vi "子界面-查看某框-只读穿透图模式.vi"(0 "框号":dbl format="%#_13g", 1 "框组":T3(array[cluster]), 2 "临界Z值":i32, 4 "临界面积百分比值":dbl, 5 "预先配置的灰度阈值":dbl, 6 "穿透图原始路径":path, 7 "部位信息":string[](array[string])=["", "34.500000", "32.500000", "1121", "34", "54.955926", "分层类", "不合格", ""], 12 "产品规格":cluster{"产品长度（周长）（mm）":dbl, "产品宽度（母线长）（mm）":dbl}) -> (14 "弥散类检测结果":string[][](table), 19 "分层类检测结果":string[][](table))   [LabVIEW 2018]
uses:
  <vilib>/vision/NI_Vision_Development_Module.lvlib
panel:
  in  "Tab Control":T1
  out "?":T2(plugin-control)
  out "Threshold Image":T2(plugin-control)
  out "Threshold Image":T2(plugin-control)
  in  "格式字符串 3":string="%f"
  in  "分隔符（'\\'代码显示） 2":string="\t"
  out "弥散和分层临界灰度值":i64
  out "弥散缺陷个数":i32
  out "分层缺陷个数":i32
  out "合格？ 弥散类":string="fencengThreshold"
  out "合格？分层类":string="fencengThreshold"
  in  "stop":bool caption="停止"
  out "弥散测量结果":dbl[][](array[numeric]) format="%.2f"
  out "?":string
  out "面积 (pixels)":i32
  in  "格式字符串 2":string="%f"
  in  "分隔符（'\\'代码显示）":string="\t"
  out "分层测量结果":dbl[][](array[numeric]) format="%.2f"
  out "缺陷初步分类的临界值":sgl format="%#.3f"
  # "所选区域信息"
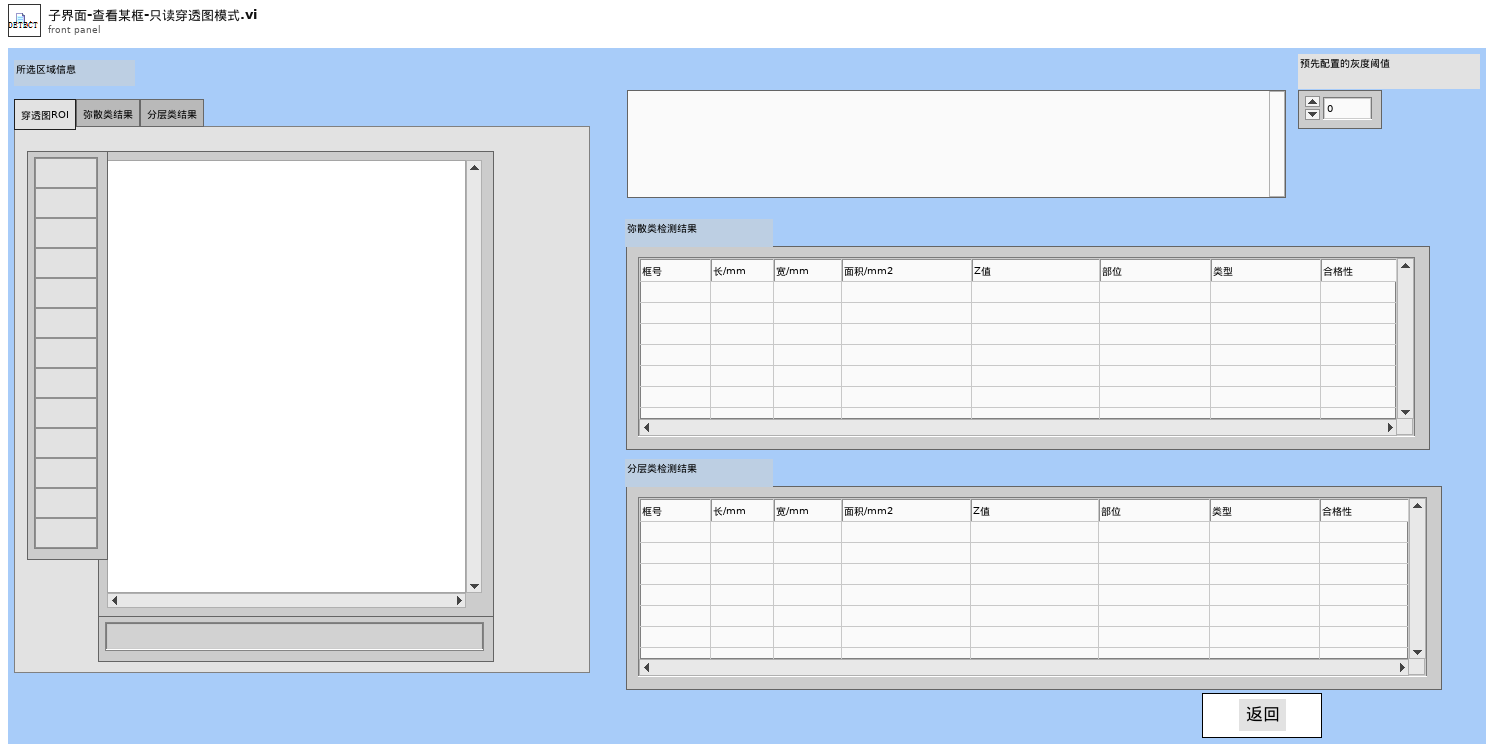
[diagram p1: front panel]
types:
  T1 = typedef "控件2.ctl" = enum32{"穿透图ROI", "弥散类结果", "分层类结果"}
  T2 = typedef "IMAQ Image.ctl" = refnum<image>
  T3 = cluster{"Global Rectangle":i32[], "Contours":cluster{"Contour Type":u32, "ROI Type":u32, "Points":i32[]}[]}[]
  T4 = typedef "Image Type" = u32
  T5 = typedef "Particle Parameters" = i32
  T6 = cluster{"Measurement Parameter":T5, "Range Lower Value":dbl, "Range Upper Value":dbl, "Range":bool, "Measurement Type":bool}[]
  T7 = cluster{"Global Rectangle":i32[], "Contours":cluster{"Contour Type":u32, "ROI Type":u32, "Points":i32[]}[]}
  T8 = cluster{"histogram":u32[], "Minimal Value":sgl, "Maximal Value":sgl, "Starting Value":sgl, "Interval Width":sgl, "Mean Value":sgl, "Standard  Variation":sgl, "Area (pixels)":i32}
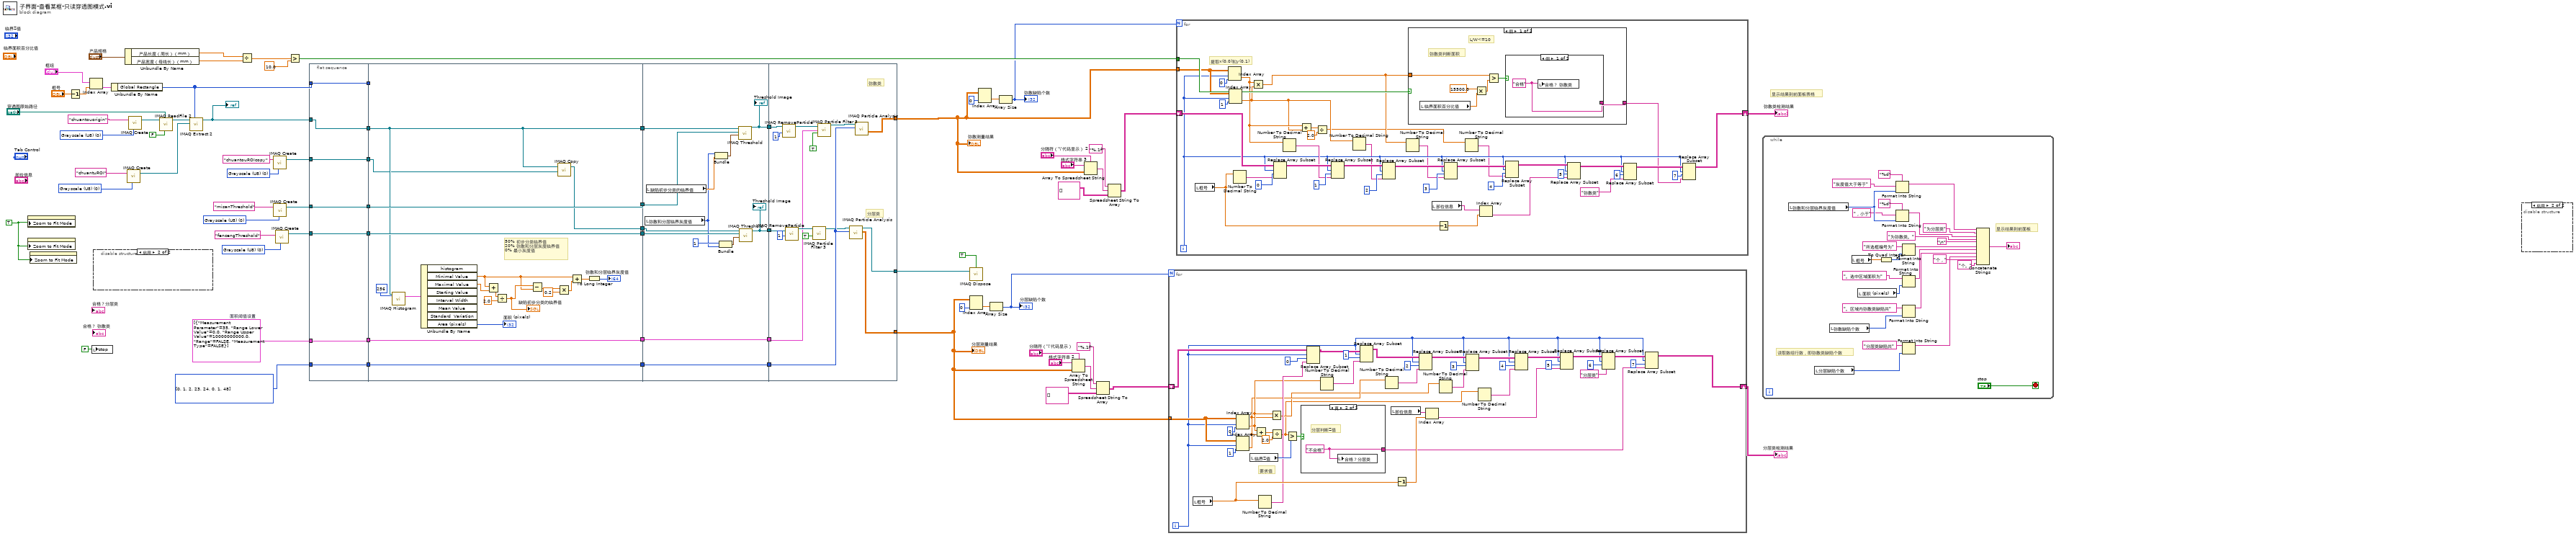
[diagram p0: block diagram]
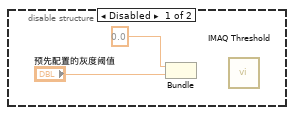
[diagram p2: hidden frame]
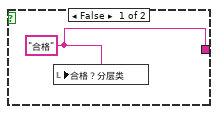
[diagram p3: hidden frame]
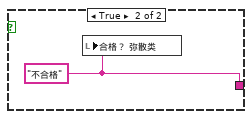
[diagram p4: hidden frame]
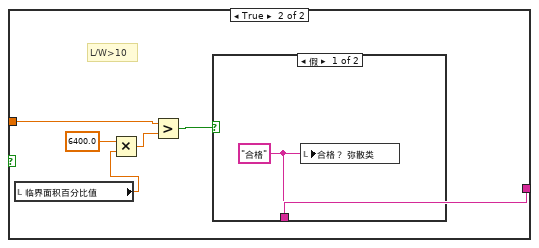
[diagram p5: hidden frame]
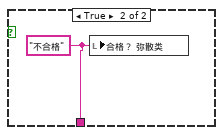
[diagram p6: hidden frame]
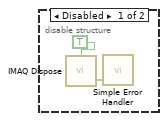
[diagram p7: hidden frame]
diagram:
  w1 = T4 0 items=["Grayscale (U8)", "Grayscale (I16)", "Grayscale (SGL)", "Complex (CSG)", "RGB (U32)", "HSL (U32)", "RGB (U64)", "Grayscale (U16)"] ("Image Type")
  w6 = TRUE ("Zoom to Fit Mode")
  w51 = T4 0 items=["Grayscale (U8)", "Grayscale (I16)", "Grayscale (SGL)", "Complex (CSG)", "RGB (U32)", "HSL (U32)", "RGB (U64)", "Grayscale (U16)"] ("Image Type")
  w52 = T4 0 items=["Grayscale (U8)", "Grayscale (I16)", "Grayscale (SGL)", "Complex (CSG)", "RGB (U32)", "HSL (U32)", "RGB (U64)", "Grayscale (U16)"] ("Image Type")
  w55 = T4 0 items=["Grayscale (U8)", "Grayscale (I16)", "Grayscale (SGL)", "Complex (CSG)", "RGB (U32)", "HSL (U32)", "RGB (U64)", "Grayscale (U16)"] ("Image Type")
  w29 = i32[] [0, 1, 2, 23, 24, 0, 1, 48] items=["Bounding Rect Width", "Bounding Rect Height", "Area"] ("Pixel Measurements")
  w33 = T6 [{"Measurement Parameter"=35, "Range Lower Value"=0.0, "Range Upper Value"=10000000000.0, "Range"=FALSE, "Measurement Type"=FALSE}]  # 面积阈值设置
  w70 = T4 0 items=["Grayscale (U8)", "Grayscale (I16)", "Grayscale (SGL)", "Complex (CSG)", "RGB (U32)", "HSL (U32)", "RGB (U64)", "Grayscale (U16)"] ("Image Type")
  # "显示结果到前面板表格"
  n1 = property class="ImageControl"("Zoom to Fit Mode"=w6) -> ()  [unwired: 2 in, 2 out]
  n2 = property class="ImageControl"("Zoom to Fit Mode"=w6) -> ()  [unwired: 2 in, 2 out]
  n3 = property class="ImageControl"("Zoom to Fit Mode"=w6) -> ()  [unwired: 2 in, 2 out]
  n4 = Decrement(x="框号") -> (x-1=w72:dbl)
  n5 = Index Array(array="框组", index=w72) -> (element=w73:T7)
  n6 = local write "stop"(FALSE ("stop")) -> ()
  n7 = disable-structure shown="启用" {
    frame Disabled {
      n8 = Bundle(0.0, "预先配置的灰度阈值"="预先配置的灰度阈值") -> ()  [unwired: 1 in, 1 out]
      n9 = call "IMAQ Threshold"() -> ()  [unwired: 6 in, 6 out]
    }
    frame Enabled {
    }
  }
  n10 = Unbundle By Name(w73) -> ("Global Rectangle"=w45:i32[])
  n11 = Unbundle By Name("产品规格") -> ("产品长度（周长）（mm）"=w63:dbl, "产品宽度（母线长）（mm）"=w62:dbl)
  n12 = call "IMAQ Create"("Image Name"="chuantuROI", "Image Type"=w55) -> ("New Image"=w54:T2)  [unwired: 3 in, 1 out]
  n13 = call "IMAQ Create"("Image Name"="chuantouorigin", "Image Type"=w70) -> ("New Image"=w57:T2)  [unwired: 3 in, 1 out]
  n14 = call "IMAQ ReadFile 2"("Use File Path Image Type"=FALSE, "File Path"="穿透图原始路径", "Image"=w57) -> ("Image Out"=w58:T2)  [unwired: 4 in, 4 out]
  n15 = call "IMAQ Extract 2"("Optional Rectangle"=w45, "Image Dst"=w54, "Image Src"=w58) -> ("Image Dst Out"=w9:T2)  [unwired: 7 in, 1 out]
  "?" <- w9
  n16 = Divide(x=w63, y=w62) -> (x/y=w66:dbl)
  n17 = call "IMAQ Create"("Image Name"="chuantouROIcopy", "Image Type"=w1) -> ("New Image"=w4:T2)  [unwired: 3 in, 1 out]
  n18 = call "IMAQ Create"("Image Name"="misanThreshold", "Image Type"=w51) -> ("New Image"=w41:T2)  [unwired: 3 in, 1 out]
  n19 = call "IMAQ Create"("Image Name"="fencengThreshold", "Image Type"=w52) -> ("New Image"=w39:T2)  [unwired: 3 in, 1 out]
  n20 = Greater?(x=w66, y=10.0) -> (0:w61:bool)
  n21 = flat-sequence {
    tunnel: w45 -> [w84]
    tunnel: w9 -> [w79]
    tunnel: [w84] -> w44
    tunnel: w41 -> [w83]
    tunnel: [w83] -> w42
    tunnel: [w82] -> w40
    tunnel: w39 -> [w82]
    tunnel: [w81] -> w34
    tunnel: w33 -> [w81]
    tunnel: [w80] -> w30
    tunnel: w29 -> [w80]
    tunnel: [w79] -> w7
    tunnel: w4 -> [w78]
    tunnel: [w78] -> w3
    tunnel: [w104] -> w43
    tunnel: [w103] -> w38
    tunnel: [w98] -> w32
    tunnel: [w97] -> w28
    tunnel: w30 -> [w97]
    tunnel: w34 -> [w98]
    tunnel: w40 -> [w103]
    tunnel: w42 -> [w104]
    tunnel: w44 -> [_]
    tunnel: [w87] -> w8
    tunnel: w7 -> [w87]
    tunnel: [w86] -> w5
    tunnel: w3 -> [w85]
    tunnel: w43 -> [w117]
    tunnel: w38 -> [w116]
    tunnel: [w106] -> w36
    tunnel: [w107] -> w35
    tunnel: w32 -> [w115]
    tunnel: [w115] -> w31
    tunnel: w28 -> [w114]
    tunnel: [w114] -> w27
    tunnel: w8 -> [w108]
    tunnel: w5 -> [w105]
    tunnel: [w129] -> w12
    tunnel: [w125] -> w20
    tunnel: [w124] -> w37
    tunnel: w36 -> [w123]
    tunnel: w35 -> [w122]
    tunnel: w31 -> [w121]
    tunnel: w27 -> [w120]
    frame #0 {
    }
    frame #1 {
      # "50% 初步分类临界值\n20% 弥散和分层灰度临界值\n0% 最小灰度值"
      n22 = call "IMAQ Histogram"("Number of Classes"=256, "Image"=w87) -> ("Histogram Report"=w101:T8)  [unwired: 8 in, 1 out]
      n23 = Unbundle By Name(w101) -> ("Minimal Value"=w89:sgl, "Maximal Value"=w95:sgl, "Area (pixels)"=→"面积 (pixels)":i32)  [unwired: 5 out]
      n24 = Add(x=w89, y=w95) -> (x+y=w94:sgl)
      n25 = Divide(x=w94, y=sgl 2.0) -> (x/y=w93:sgl)
      "缺陷初步分类的临界值" <- w93
      n26 = Subtract(x=w93, y=w89) -> (x-y=w91:sgl)
      n27 = Multiply(x=w91, y=0.2) -> (x*y=w90:dbl)
      n28 = call "IMAQ Copy"("Image Dst"=w85, "Image Src"=w87) -> ("Image Dst Out"=w86:T2)  [unwired: 4 in, 1 out]
      n29 = Add(x=w89, y=w90) -> (x+y=w88:dbl)
      n30 = To Long Integer(number=w88) -> (32bit integer=→"弥散和分层临界灰度值":i32)
    }
    frame #2 {
      n31 = local read "弥散和分层临界灰度值"() -> (w110:i64)
      n32 = local read "缺陷初步分类的临界值"() -> (w112:sgl)
      n33 = Bundle("弥散和分层临界灰度值"=w110, "缺陷初步分类的临界值"=w112) -> (w113:cluster{"弥散和分层临界灰度值":i64, "缺陷初步分类的临界值":sgl})  [unwired: 1 in]
      n34 = Bundle(1, "弥散和分层临界灰度值"=w110) -> (w109:cluster{i32, "弥散和分层临界灰度值":i64})  [unwired: 1 in]
      n35 = call "IMAQ Threshold"("Range"=w113, "Image Dst"=w117, "Image Src"=w108) -> ("Image Dst Out"=w107:T2)  [unwired: 3 in, 5 out]
      "Threshold Image" <- w107
      n36 = call "IMAQ Threshold"("Range"=w109, "Image Dst"=w116, "Image Src"=w105) -> ("Image Dst Out"=w106:T2)  [unwired: 3 in, 5 out]
      "Threshold Image" <- w106
    }
    frame #3 {
      # "分层类"
      # "弥散类"
      n37 = call "IMAQ RemoveParticle"("Number of Erosion"=1, "Image Src"=w122) -> ("Image Dst Out"=w132:T2)  [unwired: 8 in, 1 out]
      n38 = call "IMAQ RemoveParticle"("Number of Erosion"=1, "Image Src"=w123) -> ("Image Dst Out"=w128:T2)  [unwired: 8 in, 1 out]
      n39 = call "IMAQ Particle Filter 3"("Image Src"=w128, "Keep/Remove Particles (F)"=TRUE) -> ("Image Dst Out"=w118:T2)  [unwired: 11 in, 2 out]
      n40 = call "IMAQ Particle Filter 3"("Image Src"=w132, "Selection Values"=w121, "Keep/Remove Particles (F)"=TRUE) -> ("Image Dst Out"=w119:T2)  [unwired: 10 in, 2 out]
      n41 = call "IMAQ Particle Analysis"("Pixel Measurements"=w120, "Image"=w118) -> ("Particle Measurements (Pixels)"=w125:dbl[][], "Image Out (duplicate)"=w124:T2)  [unwired: 4 in, 4 out]
      n42 = call "IMAQ Particle Analysis"("Pixel Measurements"=w120, "Image"=w119) -> ("Particle Measurements (Real-World)"=w129:dbl[][])  [unwired: 4 in, 5 out]
    }
  }
  n43 = call "IMAQ Dispose"("All Images? (No)"=TRUE, "Image"=w37) -> ()  [unwired: 4 in, 1 out]
  n44 = Index Array(array=w20, index (col)=0 ("禁用的索引 (列)")) -> (element=w49:dbl[])  [unwired: 1 in]
  n45 = Index Array(array=w12, index (col)=0 ("禁用的索引 (列)")) -> (element=w47:dbl[])  [unwired: 1 in]
  n46 = Array Size(array=w49) -> (size(s)=w26:i32)
  "分层缺陷个数" <- w26
  n47 = Array Size(array=w47) -> (size(s)=w60:i32)
  "弥散缺陷个数" <- w60
  n48 = Array To Spreadsheet String(delimiter (Tab)="分隔符（'\\'代码显示）", array=w20, 3:"格式字符串 2") -> (spreadsheet string=w23:string)
  n49 = Array To Spreadsheet String(delimiter (Tab)="分隔符（'\\'代码显示） 2", array=w12, 3:"格式字符串 3") -> (spreadsheet string=w15:string)
  n50 = Spreadsheet String To Array(format string="%.1f", spreadsheet string=w23, array type (2D Dbl)=string[][] [] ("Array")) -> (array=w19:string[][])  [unwired: 1 in]
  n51 = Spreadsheet String To Array(format string="%.1f", spreadsheet string=w15, array type (2D Dbl)=string[][] [] ("Array")) -> (array=w11:string[][])  [unwired: 1 in]
  n52 = for {
    N: w26 -> [_]
    tunnel: w20 -> [w164]
    shift-right: [w142] -> w18
    shift-left: w19 -> [w153]
    i -> [w137]
    # "要求值"
    n53 = local read "框号"() -> (w162:dbl)
    n54 = Index Array(array=w164, index (row)=w137, index (col)=0 ("禁用的索引 (列)")) -> (element=w141:dbl)
    n55 = Index Array(array=w164, index (row)=w137, index (col)=1 ("禁用的索引 (列)")) -> (element=w140:dbl)
    n56 = local read "临界Z值"() -> (w170:i32)
    n57 = Add(x=w141, y=w140) -> (x+y=w171:dbl)
    n58 = Number To Decimal String(number=w162) -> (decimal integer string=w154:string)  [unwired: 1 in]
    n59 = Multiply(x=w141, y=w140) -> (x*y=w139:dbl)
    n60 = Divide(x=w171, y=2.0) -> (x/y=w136:dbl)
    n61 = Greater?(x=w136, y=w170) -> (0:w172:bool)
    n62 = case shown="真" w172 {
      tunnel: [w173 w174] -> w133
      frame False {
        w173 = "合格" ("合格？")
        n63 = local write "合格？分层类"(w173) -> ()
      }
      frame True {
        w174 = "不合格" ("合格？")
        # "分层判断Z值"
        n64 = local write "合格？分层类"(w174) -> ()
      }
    }
    n65 = Replace Array Subset(array=w153, new element=w154, index (row)=w137, index (col)=0 ("索引 (列)")) -> (w152:string[][])
    n66 = Number To Decimal String(number=w141) -> (decimal integer string=w151:string)  [unwired: 1 in]
    n67 = Replace Array Subset(array=w152, new element=w151, index (row)=w137, index (col)=1 ("索引 (列)")) -> (w149:string[][])
    n68 = Number To Decimal String(number=w140) -> (decimal integer string=w150:string)  [unwired: 1 in]
    n69 = local read "部位信息"() -> (w166:string[])
    n70 = Decrement(x=w162) -> (x-1=w165:dbl)
    n71 = Replace Array Subset(array=w149, new element=w150, index (row)=w137, index (col)=2 ("索引 (列)")) -> (w148:string[][])
    n72 = Index Array(array=w166, index=w165) -> (element=w135:string)
    n73 = Number To Decimal String(number=w139) -> (decimal integer string=w147:string)  [unwired: 1 in]
    n74 = Replace Array Subset(array=w148, new element=w147, index (row)=w137, index (col)=3 ("索引 (列)")) -> (w146:string[][])
    n75 = Number To Decimal String(number=w136) -> (decimal integer string=w138:string)  [unwired: 1 in]
    n76 = Replace Array Subset(array=w146, new element=w138, index (row)=w137, index (col)=4 ("索引 (列)")) -> (w145:string[][])
    n77 = Replace Array Subset(array=w145, new element=w135, index (row)=w137, index (col)=5 ("索引 (列)")) -> (w144:string[][])
    n78 = Replace Array Subset(array=w144, new element="分层类" ("新元素/子数组"), index (row)=w137, index (col)=6 ("索引 (列)")) -> (w143:string[][])
    n79 = Replace Array Subset(array=w143, new element=w133, index (row)=w137, index (col)=7 ("索引 (列)")) -> (w142:string[][])
  }
  "分层类检测结果" <- w18
  n80 = for {
    N: w60 -> [_]
    tunnel: w61 -> [w213]
    tunnel: w12 -> [w212]
    shift-right: [w192] -> w10
    shift-left: w11 -> [w200]
    i -> [w190]
    # "提取x(0,0)和y(0,1)"
    n81 = local read "框号"() -> (w178:dbl)
    n82 = Index Array(array=w212, index (row)=w190, index (col)=0 ("禁用的索引 (列)")) -> (element=w184:dbl)
    n83 = Index Array(array=w212, index (row)=w190, index (col)=1 ("禁用的索引 (列)")) -> (element=w183:dbl)
    n84 = Number To Decimal String(number=w178) -> (decimal integer string=w201:string)  [unwired: 1 in]
    n85 = Multiply(x=w184, y=w183) -> (x*y=w188:dbl)
    n86 = Replace Array Subset(array=w200, new element=w201, index (row)=w190, index (col)=0 ("索引 (列)")) -> (w199:string[][])
    n87 = Number To Decimal String(number=w184) -> (decimal integer string=w191:string)  [unwired: 1 in]
    n88 = Add(x=w184, y=w183) -> (x+y=w186:dbl)
    n89 = Divide(x=w186, y=2.0) -> (x/y=w182:dbl)
    n90 = Replace Array Subset(array=w199, new element=w191, index (row)=w190, index (col)=1 ("索引 (列)")) -> (w198:string[][])
    n91 = Number To Decimal String(number=w183) -> (decimal integer string=w189:string)  [unwired: 1 in]
    n92 = Replace Array Subset(array=w198, new element=w189, index (row)=w190, index (col)=2 ("索引 (列)")) -> (w197:string[][])
    n93 = Number To Decimal String(number=w188) -> (decimal integer string=w187:string)  [unwired: 1 in]
    n94 = case shown="假" w213 {
      tunnel: w188 -> [w219 w227]
      tunnel: [w217 w225] -> w175
      frame False {
        # "弥散类判断面积"
        # "L/W<=10"
        n95 = local read "临界面积百分比值"() -> (w215:dbl)
        n96 = Multiply(x=15500.0, y=w215) -> (x*y=w214:dbl)
        n97 = Greater?(x=w219, y=w214) -> (0:w218:bool)
        n98 = case shown="假" w218 {
          tunnel: [w220 w221] -> w217
          frame False {
            w220 = "合格" ("合格？")
            n99 = local write "合格？ 弥散类"(w220) -> ()
          }
          frame True {
            w221 = "不合格" ("合格？")
            n100 = local write "合格？ 弥散类"(w221) -> ()
          }
        }
      }
      frame True {
        # "L/W>10"
        n101 = local read "临界面积百分比值"() -> (w222:dbl)
        n102 = Multiply(x=6400.0, y=w222) -> (x*y=w224:dbl)
        n103 = Greater?(x=w227, y=w224) -> (0:w226:bool)
        n104 = case shown="假" w226 {
          tunnel: [w228 w229] -> w225
          frame False {
            w228 = "合格" ("合格？")
            n105 = local write "合格？ 弥散类"(w228) -> ()
          }
          frame True {
            w229 = "不合格" ("合格？")
            n106 = local write "合格？ 弥散类"(w229) -> ()
          }
        }
      }
    }
    n107 = local read "部位信息"() -> (w180:string[])
    n108 = Decrement(x=w178) -> (x-1=w179:dbl)
    n109 = Replace Array Subset(array=w197, new element=w187, index (row)=w190, index (col)=3 ("索引 (列)")) -> (w196:string[][])
    n110 = Number To Decimal String(number=w182) -> (decimal integer string=w181:string)  [unwired: 1 in]
    n111 = Index Array(array=w180, index=w179) -> (element=w177:string)
    n112 = Replace Array Subset(array=w196, new element=w181, index (row)=w190, index (col)=4 ("索引 (列)")) -> (w195:string[][])
    n113 = Replace Array Subset(array=w195, new element=w177, index (row)=w190, index (col)=5 ("索引 (列)")) -> (w194:string[][])
    n114 = Replace Array Subset(array=w194, new element="弥散类" ("新元素/子数组"), index (row)=w190, index (col)=6 ("索引 (列)")) -> (w193:string[][])
    n115 = Replace Array Subset(array=w193, new element=w175, index (row)=w190, index (col)=7 ("索引 (列)")) -> (w192:string[][])
  }
  "弥散类检测结果" <- w10
  n116 = while {
    stop <- "stop" stop-if-true
    # "显示结果到前面板"
    # "读取数组行数，即弥散类缺陷个数"
    n117 = local read "弥散和分层临界灰度值"() -> (w256:i64)
    n118 = local read "分层缺陷个数"() -> (w231:i32)
    n119 = local read "弥散缺陷个数"() -> (w230:i32)
    n120 = local read "框号"() -> (w247:dbl)
    n121 = local read "面积 (pixels)"() -> (w250:i32)
    n122 = To Quad Integer(1:w247) -> (0:w248:i64)
    n123 = Format Into String(format string="%d" ("格式字符串"), initial string="灰度值大于等于" ("初始字符串"), w256) -> (resulting string=w252:string)  [unwired: 1 in, 1 out]
    n124 = Format Into String(format string="%d" ("格式字符串"), initial string="，小于" ("初始字符串"), w256) -> (resulting string=w251:string)  [unwired: 1 in, 1 out]
    n125 = Format Into String(initial string="所选框编号为" ("初始字符串"), w248) -> (resulting string=w246:string)  [unwired: 2 in, 1 out]
    n126 = Format Into String(initial string="。选中区域面积为" ("字符串"), w250) -> (resulting string=w253:string)  [unwired: 2 in, 1 out]
    n127 = Format Into String(initial string="。区域内弥散类缺陷共" ("初始字符串"), w230) -> (resulting string=w254:string)  [unwired: 2 in, 1 out]
    n128 = Format Into String(initial string="分层类缺陷共" ("初始字符串"), w231) -> (resulting string=w255:string)  [unwired: 2 in, 1 out]
    n129 = Concatenate Strings(w252, "为分层类" ("初始字符串"), w251, "为弥散类。" ("初始字符串"), "\n", w246, w253, w254, "个，" ("字符串"), w255, "个。" ("字符串")) -> (→"?":string)
  }
  n130 = disable-structure shown="启用" {
    frame Disabled {
      n131 = call "IMAQ Dispose"("All Images? (No)"=TRUE) -> ("error out"=w258:errorcluster)  [unwired: 5 in]
      n132 = call <vilib>:"Simple Error Handler.vi"("error in (no error)"=w258) -> ()  [unwired: 4 in, 5 out]
    }
    frame Enabled {
    }
  }
  "分层测量结果" <- w20
  "弥散测量结果" <- w12
